vi "Launcher.vi"   [LabVIEW 2020]
uses:
  BLE_Request.ctl
  BLE_Request_Command.ctl
  Controller_Response.ctl
  Controller_Response_Command.ctl
  Controller_Request.ctl
  Controller_Request_Command.ctl
types:
  T1 = typedef "Controller_Request.ctl" = cluster{"Command":T2, "Parameter":variant}
  T2 = typedef "Controller_Request_Command.ctl" = enum16{"BLE_ScannedDevices", "BLE_ConnectionResult", "BLE_NotificationToogleResult", "BLE_NotificationData", "BLE_ConnTimeout", "BLE_CloseResult", "User_Init", "User_ScanRequest", "User_ConnectionRequest", "User_CloseRequest", "User_NotficationToggleRequest"}
  T3 = typedef "BLE_Request.ctl" = cluster{"Command":T4, "Parameter":variant}
  T4 = typedef "BLE_Request_Command.ctl" = enum16{"BLE_Idle", "BLE_Init", "BLE_ScanToogle", "BLE_Connect", "BLE_NotificationToogle", "BLE_Close"}
  T5 = typedef "Controller_Response.ctl" = cluster{"Command":T6, "Parameter":variant}
  T6 = typedef "Controller_Response_Command.ctl" = enum16{"Init", "ScanResult", "ConnectionResult", "ConnectionTimeout", "NotificationToogleResult", "NotificationData", "CloseResult"}
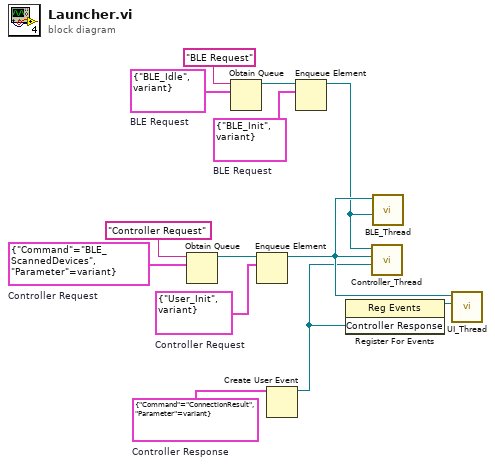
[diagram p0: block diagram]
diagram:
  w5 = T1 {"Command"=enum."User_Init", "Parameter"=variant}  # Controller Request
  w9 = T1 {"Command"=enum."BLE_ScannedDevices", "Parameter"=variant}  # Controller Request
  w7 = T3 {"Command"=enum."BLE_Init", "Parameter"=variant}  # BLE Request
  w8 = T5 {"Command"=enum."ConnectionResult", "Parameter"=variant}  # Controller Response
  w12 = T3 {"Command"=enum."BLE_Idle", "Parameter"=variant}  # BLE Request
  n1 = Obtain Queue(name (unnamed)="Controller Request", element data type=w9) -> (queue out=w6:refnum<queue>)  [unwired: 3 in, 2 out]
  n2 = Obtain Queue(name (unnamed)="BLE Request", element data type=w12) -> (queue out=w11:refnum<queue>)  [unwired: 3 in, 2 out]
  n3 = Enqueue Element(queue=w6, element=w5) -> (queue out=w4:refnum<queue>)  [unwired: 2 in, 2 out]
  n4 = Create User Event(user event datatype=w8) -> (user event=w1:refnum<user-event>)  [unwired: 1 in, 1 out]
  n5 = Enqueue Element(queue=w11, element=w7) -> (queue out=w3:refnum<queue>)  [unwired: 2 in, 2 out]
  n6 = register-events(w1) -> (reference out=w2:refnum<event-registration>)  [unwired: 2 in, 1 out]
  n7 = call "Controller_Thread.vi"("user event"=w1, "controller queue in"=w4, "ble queue out"=w3) -> ()  [unwired: 9 in]
  n8 = call "BLE_Thread.vi"("ble queue in"=w3, "controller queue out"=w4) -> ()  [unwired: 10 in]
  n9 = call "UI_Thread.vi"("Event Registration Refnum"=w2, "controller queue out"=w4) -> ()  [unwired: 10 in]
